vi "ConvertTextBasedCodeToLabVIEW_CreateMissingClassesDefinition.vi"(8 "error in (no error)":errorcluster, 10 "Action":T1[](array[typedef]), 11 "ClassName":string[](array[string])) -> (0 "error out":errorcluster, 3 "Classes":T2[](array[typedef]))   [LabVIEW 2020]
uses:
  <resource>/Framework/Providers/Open_GDS/ClassProviders/Common/String/GDSString_ClassDescriptionType.ctl
  <resource>/Framework/Providers/Open_GDS/ClassProviders/Common/String/GDSString_AccessScopeModifierType.ctl
  <resource>/Framework/Providers/Open_GDS/ClassProviders/Common/String/GDSString_ModifierType.ctl
  <resource>/Framework/Providers/Open_GDS/ClassProviders/Common/String/GDSString_MethodDescriptionType.ctl
  <resource>/Framework/Providers/Open_GDS/ClassProviders/Common/CommonVIs/CommonVIs_AttributeType.ctl
  <resource>/Framework/Providers/Open_GDS/ClassProviders/Common/CommonVIs/CommonVIs_AttributeDataType.ctl
  <resource>/Framework/Providers/Open_GDS/ClassProviders/Common/CommonVIs/CommonVIs_PropertyType.ctl
  <resource>/Framework/Providers/Open_GDS/ClassProviders/Common/String/GDSString_ClassParentType.ctl
  <resource>/Framework/Providers/Open_GDS/ClassProviders/Common/String/GDSString_ClassType.ctl
  <resource>/Framework/Providers/Open_GDS/ClassProviders/Common/String/GDSString_ClassOwnerType.ctl
  <resource>/Framework/Providers/Open_GDS/ClassProviders/Common/CommonVIs/CommonVIs_EnumType.ctl
  <resource>/Framework/Providers/Open_GDS/ClassProviders/Common/CommonVIs/CommonVIs_StructType.ctl
  <resource>/Framework/Providers/Open_GDS/ClassProviders/Common/ConvertTextToLv_SubVIs/ConvertTextBasedCodeToLabVIEW_MissingTypeOptions.ctl
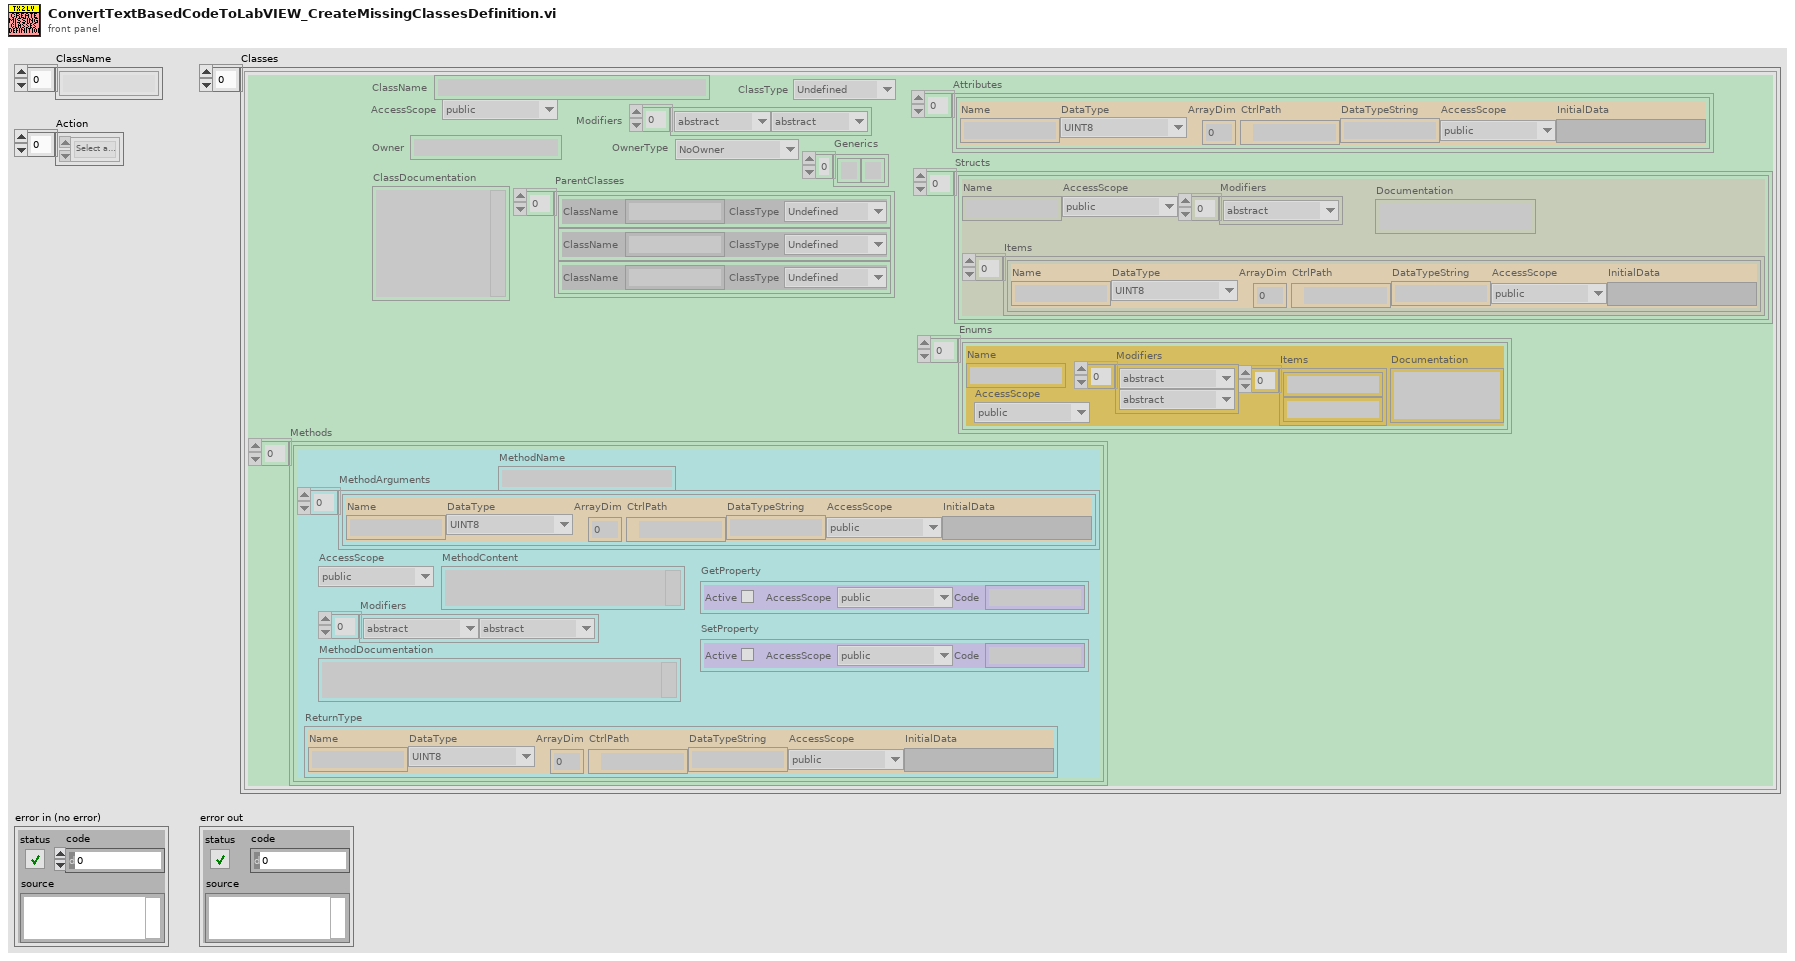
[diagram p1: front panel]
types:
  T1 = typedef "ConvertTextBasedCodeToLabVIEW_MissingTypeOptions.ctl" = enum16{"Select action to handle missing type", "Create stub code as class", "Create stub code as interface", "Remove dependency to this type"}
  T2 = typedef "GDSString_ClassDescriptionType.ctl" = cluster{"ClassName":string, "AccessScope":T3, "Modifiers":T4[], "ClassDocumentation":string, "Methods":T5[], "ParentClasses":T9[], "ClassType":T10, "Owner":string, "OwnerType":T11, "Generics":string[], "Attributes":T6[], "Enums":T12[], "Structs":T13[]}
  T3 = typedef "GDSString_AccessScopeModifierType.ctl" = enum16{"public", "private", "protected", "internal"}
  T4 = typedef "GDSString_ModifierType.ctl" = enum16{"abstract", "static", "final", "synchronized", "strictfp", "async", "const", "event", "extern", "new", "native ", "override", "partial", "readonly", "sealed", "unsafe", "virtual", "volatile"}
  T5 = typedef "GDSString_MethodDescriptionType.ctl" = cluster{"ReturnType":T6, "MethodName":string, "AccessScope":T3, "Modifiers":T4[], "MethodDocumentation":string, "MethodContent":string, "MethodArguments":T6[], "GetProperty":T8, "SetProperty":T8}
  T6 = typedef "CommonVIs_AttributeType.ctl" = cluster{"Name":string, "DataType":T7, "ArrayDim":i32, "CtrlPath":path, "DataTypeString":string, "AccessScope":T3, "InitialData":variant}
  T7 = typedef "CommonVIs_AttributeDataType.ctl" = enum16{"UINT8", "INT8", "UINT16", "INT16", "UINT32", "INT32", "UINT64", "INT64", "SGL", "DBL", "EXT", "CSG", "CDB", "CXT", "TimeStamp", "STRING", "PATH", "BOOL", "ENUM", "RefNum", "VIRefNum", "LabVIEW Class", "Cluster", "Variant", "TypeDef", "Waveform", "LabVIEW Object", "Other", "void"}
  T8 = typedef "CommonVIs_PropertyType.ctl" = cluster{"Active":bool, "AccessScope":T3, "Code":string}
  T9 = typedef "GDSString_ClassParentType.ctl" = cluster{"ClassName":string, "ClassType":T10}
  T10 = typedef "GDSString_ClassType.ctl" = enum16{"Undefined", "Class", "Interface"}
  T11 = typedef "GDSString_ClassOwnerType.ctl" = enum16{"NoOwner", "Class", "Package/NameSpace"}
  T12 = typedef "CommonVIs_EnumType.ctl" = cluster{"Name":string, "AccessScope":T3, "Modifiers":T4[], "Items":string[], "Documentation":string}
  T13 = typedef "CommonVIs_StructType.ctl" = cluster{"Name":string, "AccessScope":T3, "Modifiers":T4[], "Items":T6[], "Documentation":string}
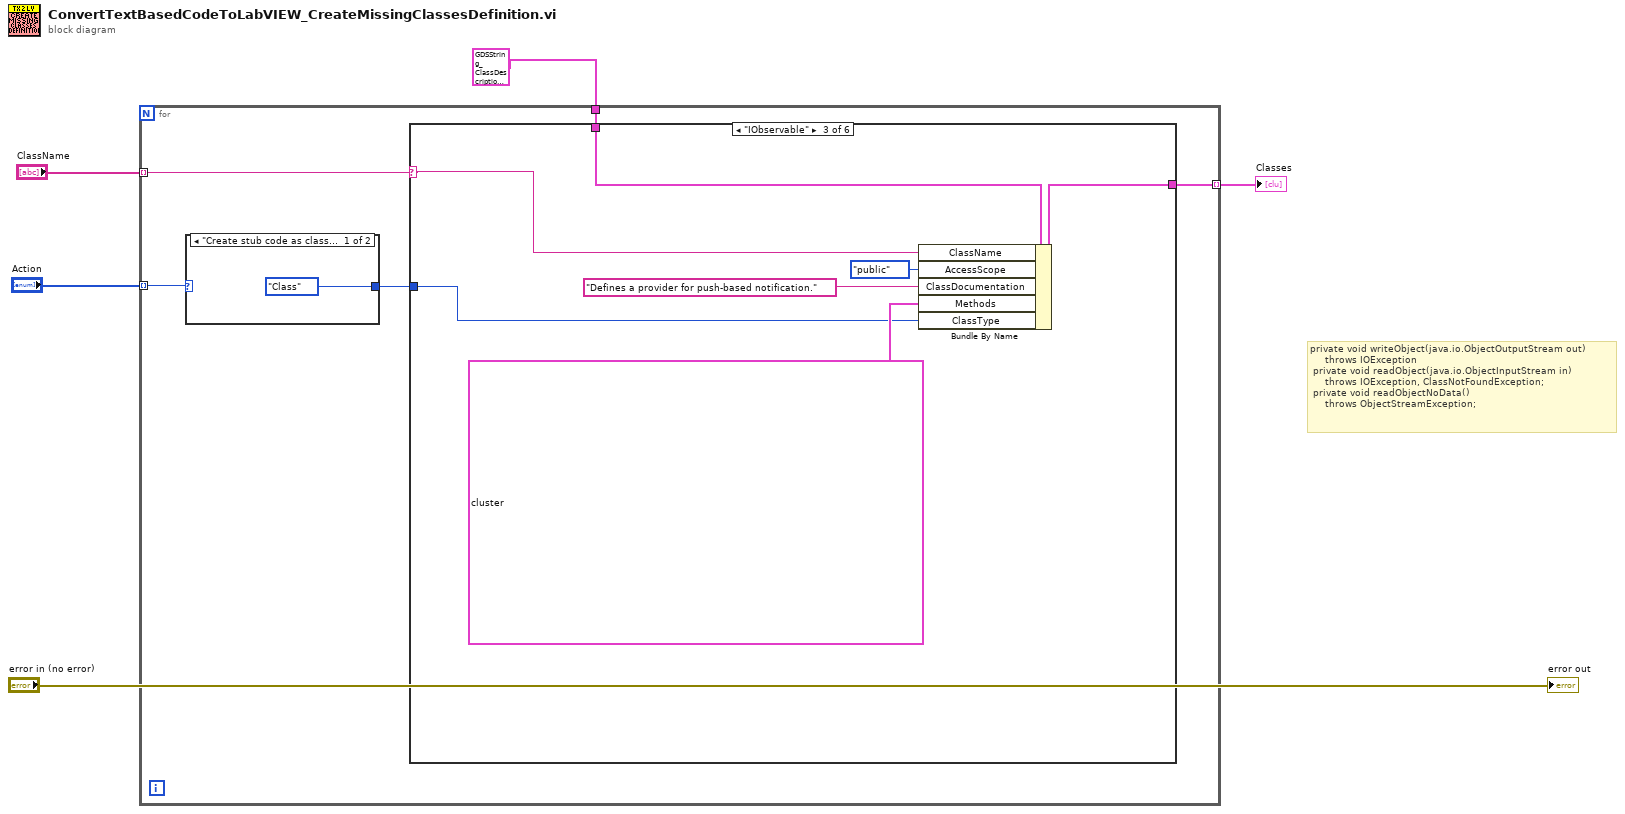
[diagram p0: block diagram]
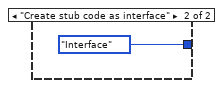
[diagram p2: hidden frame]
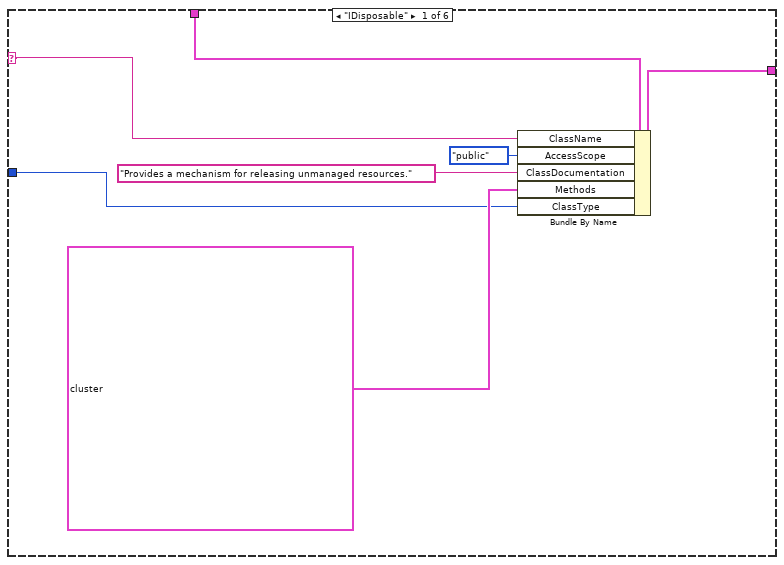
[diagram p3: hidden frame]
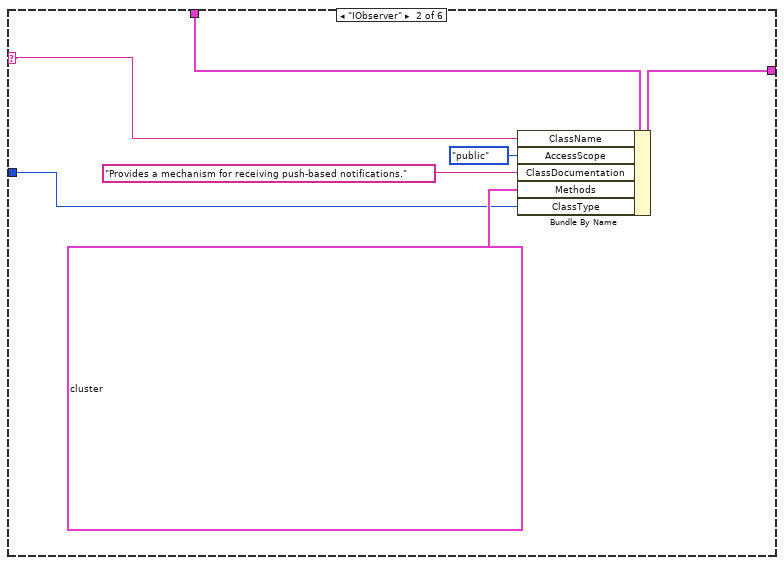
[diagram p4: hidden frame]
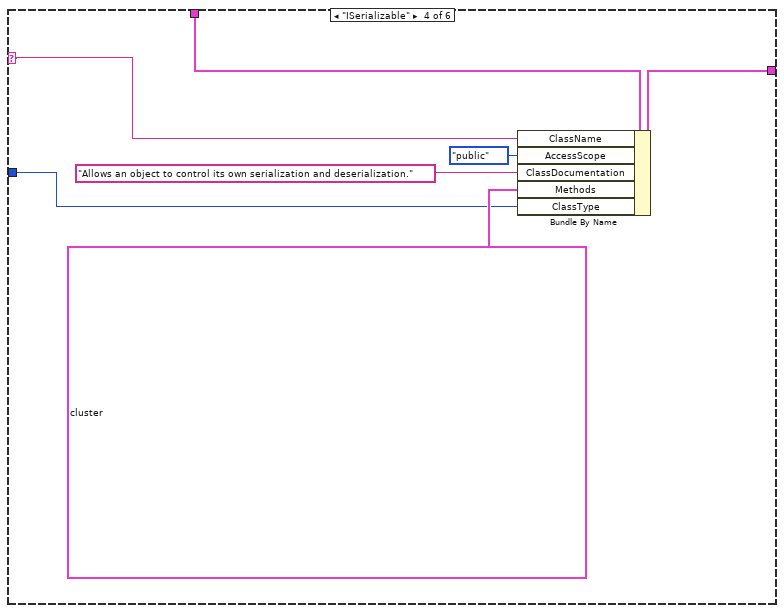
[diagram p5: hidden frame]
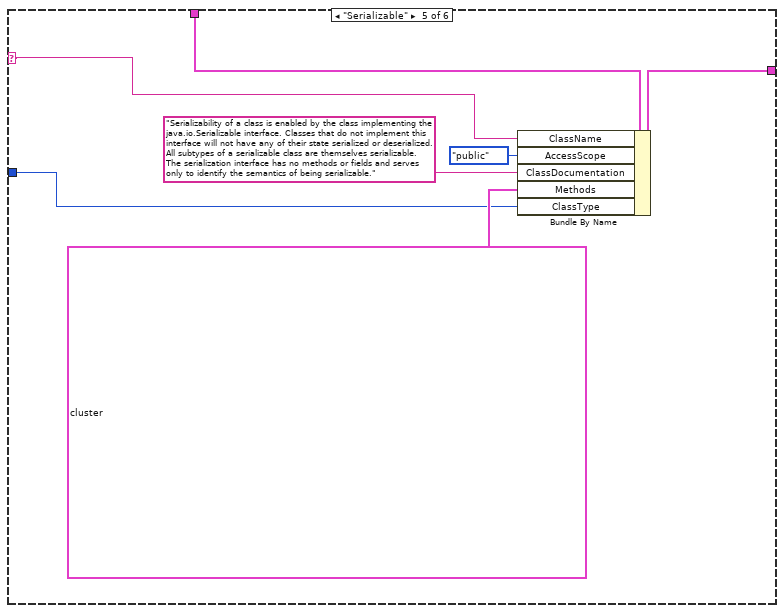
[diagram p6: hidden frame]
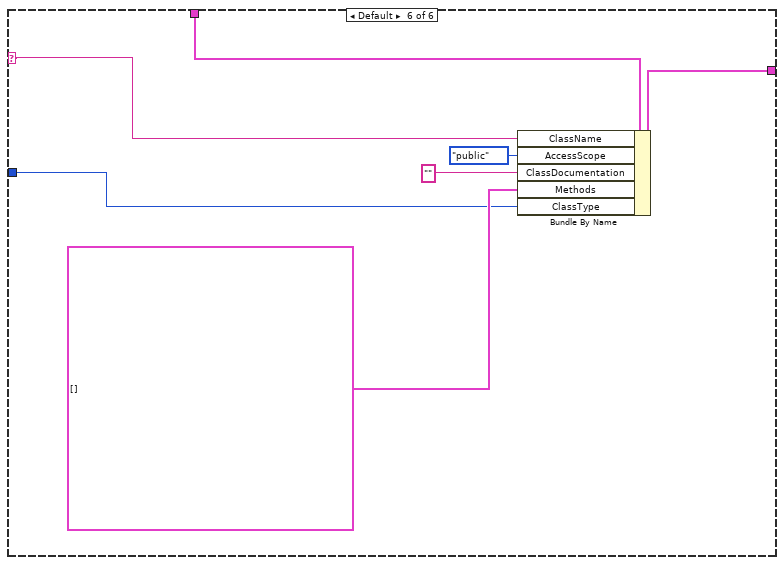
[diagram p7: hidden frame]
diagram:
  # "private void writeObject(java.io.ObjectOutputStream out)\n     throws IOException\n private void readObject(java.io.ObjectInputStream in)\n     throws IOException, ClassNotFoundException;\n private void readObjectNoData()\n     throws ObjectStreamException;"
  n1 = for {
    tunnel: "ClassName" -> [w10] mode=indexing
    tunnel: T2 {"ClassName"="", "AccessScope"=enum."public", "Modifiers"=[], "ClassDocumentation"="", "Methods"=[], "ParentClasses"=[], "ClassType"=enum."Undefined", "Owner"="", "OwnerType"=enum."NoOwner", "Generics"=[], "Attributes"=[], "Enums"=[], "Structs"=[]} ("Class") -> [w9]
    tunnel: "Action" -> [w8] mode=indexing
    tunnel: [w6] -> w1 mode=indexing
    n2 = case shown="\"Create stub code as class\", Default" w8 {
      tunnel: [GDSString_ClassType."Class" ("ClassType") GDSString_ClassType."Interface" ("ClassType")] -> w7
      frame "Create stub code as class", Default {
      }
      frame "Create stub code as interface" {
      }
    }
    n3 = case shown="\"IObservable\"" w10 {
      selector: w10 -> [w18 w25 w32 w39 w41 w53]
      tunnel: w9 -> [w19 w26 w33 w40 w47 w54]
      tunnel: w7 -> [w14 w21 w28 w35 w43 w49]
      tunnel: [w13 w20 w27 w34 w42 w48] -> w6
      frame "IDisposable" {
        n4 = Bundle By Name(cluster=w19, "ClassName"=w18, "AccessScope"=GDSString_AccessScopeModifierType."public", "ClassDocumentation"="Provides a mechanism for releasing unmanaged resources.", "Methods"=T5[] [{"ReturnType"={"Name"="", "DataType"=enum."void", "ArrayDim"=0, "CtrlPath"=path "", "DataTypeString"="", "AccessScope"=enum."public", "InitialData"=variant}, "MethodName"="Dispose", "AccessScope"=enum."public", "Modifiers"=[], "MethodDocumentation"="Performs application-defined tasks associated with freeing, releasing, or resetting unmanaged resources", "MethodContent"="", "MethodArguments"=[], "GetProperty"={"Active"=FALSE, "AccessScope"=enum."public", "Code"=""}, "SetProperty"={"Active"=FALSE, "AccessScope"=enum."public", "Code"=""}}], "ClassType"=w14) -> (w13:T2)
      }
      frame "IObserver" {
        n5 = Bundle By Name(cluster=w26, "ClassName"=w25, "AccessScope"=GDSString_AccessScopeModifierType."public", "ClassDocumentation"="Provides a mechanism for receiving push-based notifications.", "Methods"=T5[] [{"ReturnType"={"Name"="", "DataType"=enum."void", "ArrayDim"=0, "CtrlPath"=path "", "DataTypeString"="", "AccessScope"=enum."public", "InitialData"=variant}, "MethodName"="OnCompleted", "AccessScope"=enum."public", "Modifiers"=[], "MethodDocumentation"="Notifies the observer that the provider has finished sending push-based notifications.", "MethodContent"="", "MethodArguments"=[], "GetProperty"={"Active"=FALSE, "AccessScope"=enum."public", "Code"=""}, "SetProperty"={"Active"=FALSE, "AccessScope"=enum."public", "Code"=""}}, {"ReturnType"={"Name"="", "DataType"=enum."void", "ArrayDim"=0, "CtrlPath"=path "", "DataTypeString"="", "AccessScope"=enum."public", "InitialData"=variant}, "MethodName"="OnError", "AccessScope"=enum."public", "Modifiers"=[], "MethodDocumentation"="Notifies the observer that the provider has experienced an error condition.", "MethodContent"="", "MethodArguments"=[{"Name"="Error", "DataType"=enum."Variant", "ArrayDim"=0, "CtrlPath"=path "", "DataTypeString"="Exception", "AccessScope"=enum."public", "InitialData"=variant}], "GetProperty"={"Active"=FALSE, "AccessScope"=enum."public", "Code"=""}, "SetProperty"={"Active"=FALSE, "AccessScope"=enum."public", "Code"=""}}, {"ReturnType"={"Name"="", "DataType"=enum."void", "ArrayDim"=0, "CtrlPath"=path "", "DataTypeString"="", "AccessScope"=enum."public", "InitialData"=variant}, "MethodName"="OnNext", "AccessScope"=enum."public", "Modifiers"=[], "MethodDocumentation"="Provides the observer with new data.", "MethodContent"="", "MethodArguments"=[{"Name"="Value", "DataType"=enum."Variant", "ArrayDim"=0, "CtrlPath"=path "", "DataTypeString"="", "AccessScope"=enum."public", "InitialData"=variant}], "GetProperty"={"Active"=FALSE, "AccessScope"=enum."public", "Code"=""}, "SetProperty"={"Active"=FALSE, "AccessScope"=enum."public", "Code"=""}}], "ClassType"=w21) -> (w20:T2)
      }
      frame "IObservable" {
        n6 = Bundle By Name(cluster=w33, "ClassName"=w32, "AccessScope"=GDSString_AccessScopeModifierType."public", "ClassDocumentation"="Defines a provider for push-based notification.", "Methods"=T5[] [{"ReturnType"={"Name"="", "DataType"=enum."LabVIEW Class", "ArrayDim"=0, "CtrlPath"=path "", "DataTypeString"="IDisposable", "AccessScope"=enum."public", "InitialData"=variant}, "MethodName"="Subscribe", "AccessScope"=enum."public", "Modifiers"=[], "MethodDocumentation"="Notifies the provider that an observer is to receive notifications.", "MethodContent"="", "MethodArguments"=[{"Name"="observer", "DataType"=enum."Variant", "ArrayDim"=0, "CtrlPath"=path "", "DataTypeString"="", "AccessScope"=enum."public", "InitialData"=variant}], "GetProperty"={"Active"=FALSE, "AccessScope"=enum."public", "Code"=""}, "SetProperty"={"Active"=FALSE, "AccessScope"=enum."public", "Code"=""}}], "ClassType"=w28) -> (w27:T2)
      }
      frame "ISerializable" {
        n7 = Bundle By Name(cluster=w40, "ClassName"=w39, "AccessScope"=GDSString_AccessScopeModifierType."public", "ClassDocumentation"="Allows an object to control its own serialization and deserialization.", "Methods"=T5[] [{"ReturnType"={"Name"="", "DataType"=enum."void", "ArrayDim"=0, "CtrlPath"=path "", "DataTypeString"="", "AccessScope"=enum."public", "InitialData"=variant}, "MethodName"="GetObjectData", "AccessScope"=enum."public", "Modifiers"=[], "MethodDocumentation"="Populates a SerializationInfo with the data needed to serialize the target object.", "MethodContent"="", "MethodArguments"=[{"Name"="info", "DataType"=enum."Variant", "ArrayDim"=0, "CtrlPath"=path "", "DataTypeString"="SerializationInfo", "AccessScope"=enum."public", "InitialData"=variant}, {"Name"="context", "DataType"=enum."Variant", "ArrayDim"=0, "CtrlPath"=path "", "DataTypeString"="StreamingContext ", "AccessScope"=enum."public", "InitialData"=variant}], "GetProperty"={"Active"=FALSE, "AccessScope"=enum."public", "Code"=""}, "SetProperty"={"Active"=FALSE, "AccessScope"=enum."public", "Code"=""}}], "ClassType"=w35) -> (w34:T2)
      }
      frame "Serializable" {
        n8 = Bundle By Name(cluster=w47, "ClassName"=w41, "AccessScope"=GDSString_AccessScopeModifierType."public", "ClassDocumentation"="Serializability of a class is enabled by the class implementing the java.io.Serializable interface. Classes that do not implement this interface will not have any of their state serialized or deserialized. All subtypes of a serializable class are themselves serializable. The serialization interface has no methods or fields and serves only to identify the semantics of being serializable.", "Methods"=T5[] [{"ReturnType"={"Name"="", "DataType"=enum."void", "ArrayDim"=0, "CtrlPath"=path "", "DataTypeString"="", "AccessScope"=enum."public", "InitialData"=variant}, "MethodName"="writeObject", "AccessScope"=enum."public", "Modifiers"=[], "MethodDocumentation"="Populates a SerializationInfo with the data needed to serialize the target object.", "MethodContent"="", "MethodArguments"=[{"Name"="out", "DataType"=enum."Variant", "ArrayDim"=0, "CtrlPath"=path "", "DataTypeString"="ObjectOutputStream", "AccessScope"=enum."public", "InitialData"=variant}], "GetProperty"={"Active"=FALSE, "AccessScope"=enum."public", "Code"=""}, "SetProperty"={"Active"=FALSE, "AccessScope"=enum."public", "Code"=""}}, {"ReturnType"={"Name"="", "DataType"=enum."void", "ArrayDim"=0, "CtrlPath"=path "", "DataTypeString"="", "AccessScope"=enum."public", "InitialData"=variant}, "MethodName"="readObject", "AccessScope"=enum."public", "Modifiers"=[], "MethodDocumentation"="", "MethodContent"="", "MethodArguments"=[{"Name"="in", "DataType"=enum."Variant", "ArrayDim"=0, "CtrlPath"=path "", "DataTypeString"="ObjectInputStream", "AccessScope"=enum."public", "InitialData"=variant}], "GetProperty"={"Active"=FALSE, "AccessScope"=enum."public", "Code"=""}, "SetProperty"={"Active"=FALSE, "AccessScope"=enum."public", "Code"=""}}, {"ReturnType"={"Name"="", "DataType"=enum."void", "ArrayDim"=0, "CtrlPath"=path "", "DataTypeString"="", "AccessScope"=enum."public", "InitialData"=variant}, "MethodName"="readObjectNoData", "AccessScope"=enum."public", "Modifiers"=[], "MethodDocumentation"="", "MethodContent"="", "MethodArguments"=[], "GetProperty"={"Active"=FALSE, "AccessScope"=enum."public", "Code"=""}, "SetProperty"={"Active"=FALSE, "AccessScope"=enum."public", "Code"=""}}], "ClassType"=w43) -> (w42:T2)
      }
      frame Default {
        n9 = Bundle By Name(cluster=w54, "ClassName"=w53, "AccessScope"=GDSString_AccessScopeModifierType."public", "ClassDocumentation"="", "Methods"=T5[] [], "ClassType"=w49) -> (w48:T2)
      }
    }
  }
  "Classes" <- w1
  "error out" <- "error in (no error)"
